vi "BITMAPFILEHEADER.vi"(11 "图像维数":i32[](array[numeric])) -> (3 "位图文件头":u8[](array[numeric]))   [LabVIEW 2012]
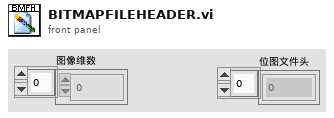
[diagram p1: front panel]
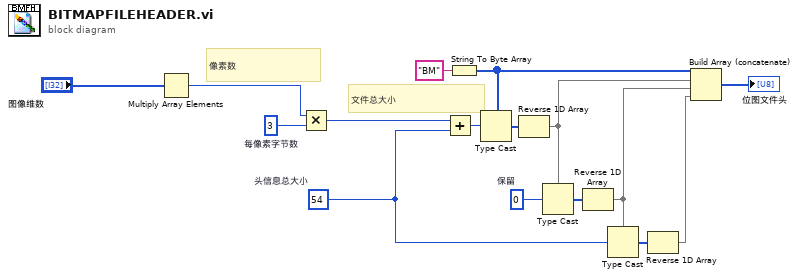
[diagram p0: block diagram]
diagram:
  w16 = 54  # 头信息总大小
  w15 = 0  # 保留
  w10 = 3  # 每像素字节数
  # "文件总大小"
  # "像素数"
  n1 = Multiply Array Elements ("数组元素相乘")(1:"图像维数") -> (0:w13:i32)
  n2 = Multiply ("乘")(x=w13, y=w10) -> (x*y=w1:i32)
  n3 = Add ("加")(x=w1, y=w16) -> (x+y=w8:i32)
  n4 = String To Byte Array ("字符串至字节数组转换")(string="BM") -> (unsigned byte array=w9:u8[])
  n5 = Type Cast ("强制类型转换")(type=w9, x=w8) -> (*(type *) &x=w7:u8[])
  n6 = Reverse 1D Array ("反转一维数组")(array=w7) -> (reversed array=w6:u8[])
  n7 = Type Cast ("强制类型转换")(type=w6, x=w15) -> (*(type *) &x=w5:u8[])
  n8 = Reverse 1D Array ("反转一维数组")(array=w5) -> (reversed array=w4:u8[])
  n9 = Type Cast ("强制类型转换")(type=w4, x=w16) -> (*(type *) &x=w2:u8[])
  n10 = Reverse 1D Array ("反转一维数组")(array=w2) -> (reversed array=w3:u8[])
  n11 = Build Array (concatenate) ("创建数组")(w9, w6, w4, w3) -> (→"位图文件头":u8[])
